vi "LV SciSDK FRAME SINGLE.vi"(7 "Frame Handle In":T3, 9 "Board Handle In":T1, 11 "error in (no error)":errorcluster) -> (4 "NI Error Code":i32, 6 "Frame Buffer Out":T2, 8 "Frame Handle Out":T3, 10 "Board Handle Out":T1, 15 "error out":errorcluster)   [LabVIEW 2021, in "SciSDK_Labview.lvlib"]
doc: "You need this VI to read a single time data from a frame component"
uses:
  SciSDK_Labview.lvlib
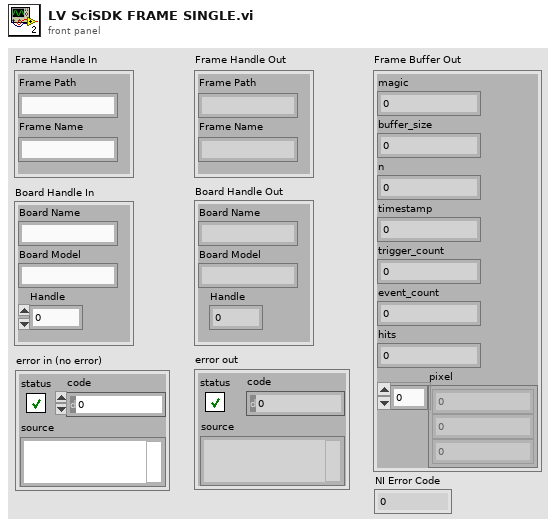
[diagram p1: front panel]
types:
  T1 = cluster{"Board Name":string, "Board Model":string, "Handle":u64}
  T2 = cluster{"magic":u32, "buffer_size":u32, "n":u64, "timestamp":u64, "trigger_count":u64, "event_count":u64, "hits":u64, "pixel":u32[]}
  T3 = cluster{"Frame Path":string, "Frame Name":string}
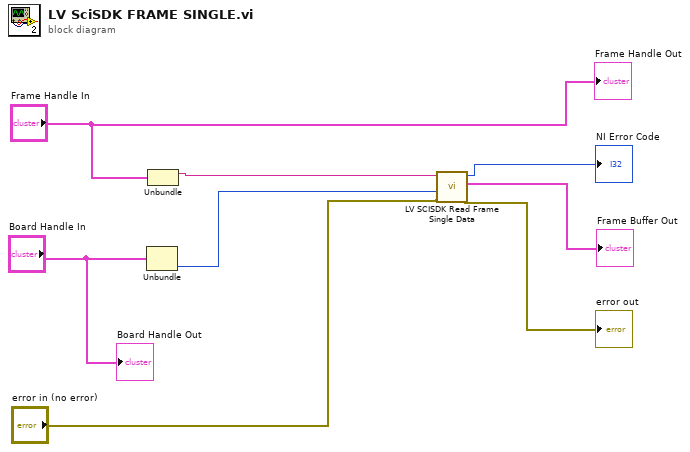
[diagram p0: block diagram]
diagram:
  n1 = Unbundle("Board Handle In") -> ("Handle"=w2:u64)  [unwired: 2 out]
  n2 = Unbundle("Frame Handle In") -> ("Frame Path"=w1:string)  [unwired: 1 out]
  n3 = call "LV SCISDK Read Frame Single Data.vi"("Path"=w1, "handle"=w2, "error in (no error)"="error in (no error)") -> ("function return"=→"NI Error Code":i32, "buffer out"=→"Frame Buffer Out":T2, "error out"=→"error out":errorcluster)  [unwired: 4 in, 1 out]
  "Frame Handle Out" <- "Frame Handle In"
  "Board Handle Out" <- "Board Handle In"
